vi "Project (1).vi"() -> ()   [LabVIEW 2023]
uses:
  <vilib>/Utility/file.llb/Read Delimited Spreadsheet (string).vi
  <instrlib>/Agilent N934X Series/Agilent N934X Series.lvlib
  System.Windows.Forms
panel:
  out "loop#":i32
  out "size(s)":i32
  out "Trace Data":dbl[](array[numeric])
  in  "Measurement Mode (0: Off)":i32(ring) items=["Off", "Channel Power Measurement", "Adjacent Channel Power Ratio Measurement", "Occupied Bandwidth Measurement", "Spectrum Monitor", "Spectrum Emission Mask", "Channel Scanner", "AM Measurement", "ASK Measurement", "FM Measurement", "FSK Measurement"]
  in  "Measurement Type (0: Spectrum Analyzer)":i32(ring) items=["Spectrum Analyzer", "Tracking Generator", "Power Meter", "Modulation Analyzer", "Reflection Measurement"]
  out "Instrument Firmware Revision":string
  out "Instrument Driver Revision":string
  in  "VISA resource name":refnum<visa-resource-name>
  in  "jkjk":bool
  out "jkjk":string
  out "jkjk":string
  out "jkjk":string
  in  "jkjk":bool
  in  "Tab Control":T1(tab)
  in  "?":bool
  out "?":string
  out "Step:":i32
  in  "Start Frequency (MHz)":dbl
  in  "IIM":bool
  in  "Stop Frequency (MHz)":dbl
  in  "Length of Cable (ft)":dbl
  in  "Cable Attenuation (dB/ft)":dbl
  in  "Velocity Factor (%)":dbl
  out "Waveform Graph":dbl[](graph)
  in  "?":refnum<k24>(container)
  out "Section:":string
  # "VSWR and Distance to Fault Test"
  # "For a single carrier"
  # "(LBand TX)  +  LBand RX = 2475 MHz"
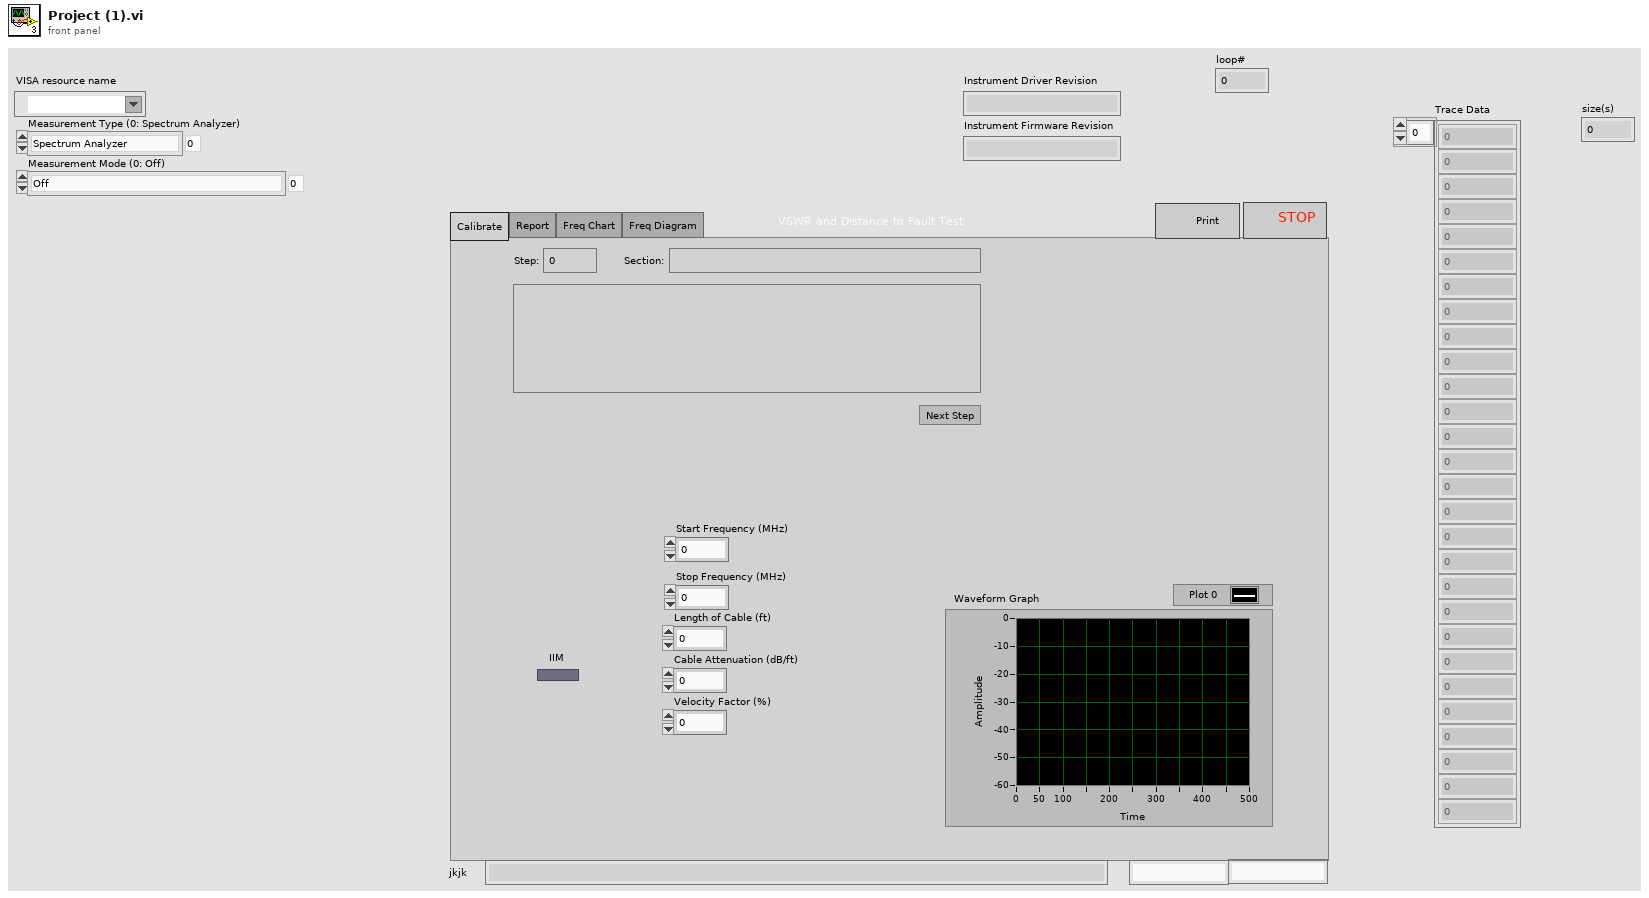
[diagram p1: front panel]
types:
  T1 = enum32{"Calibrate", "Report", "Freq Chart", "Freq Diagram"}
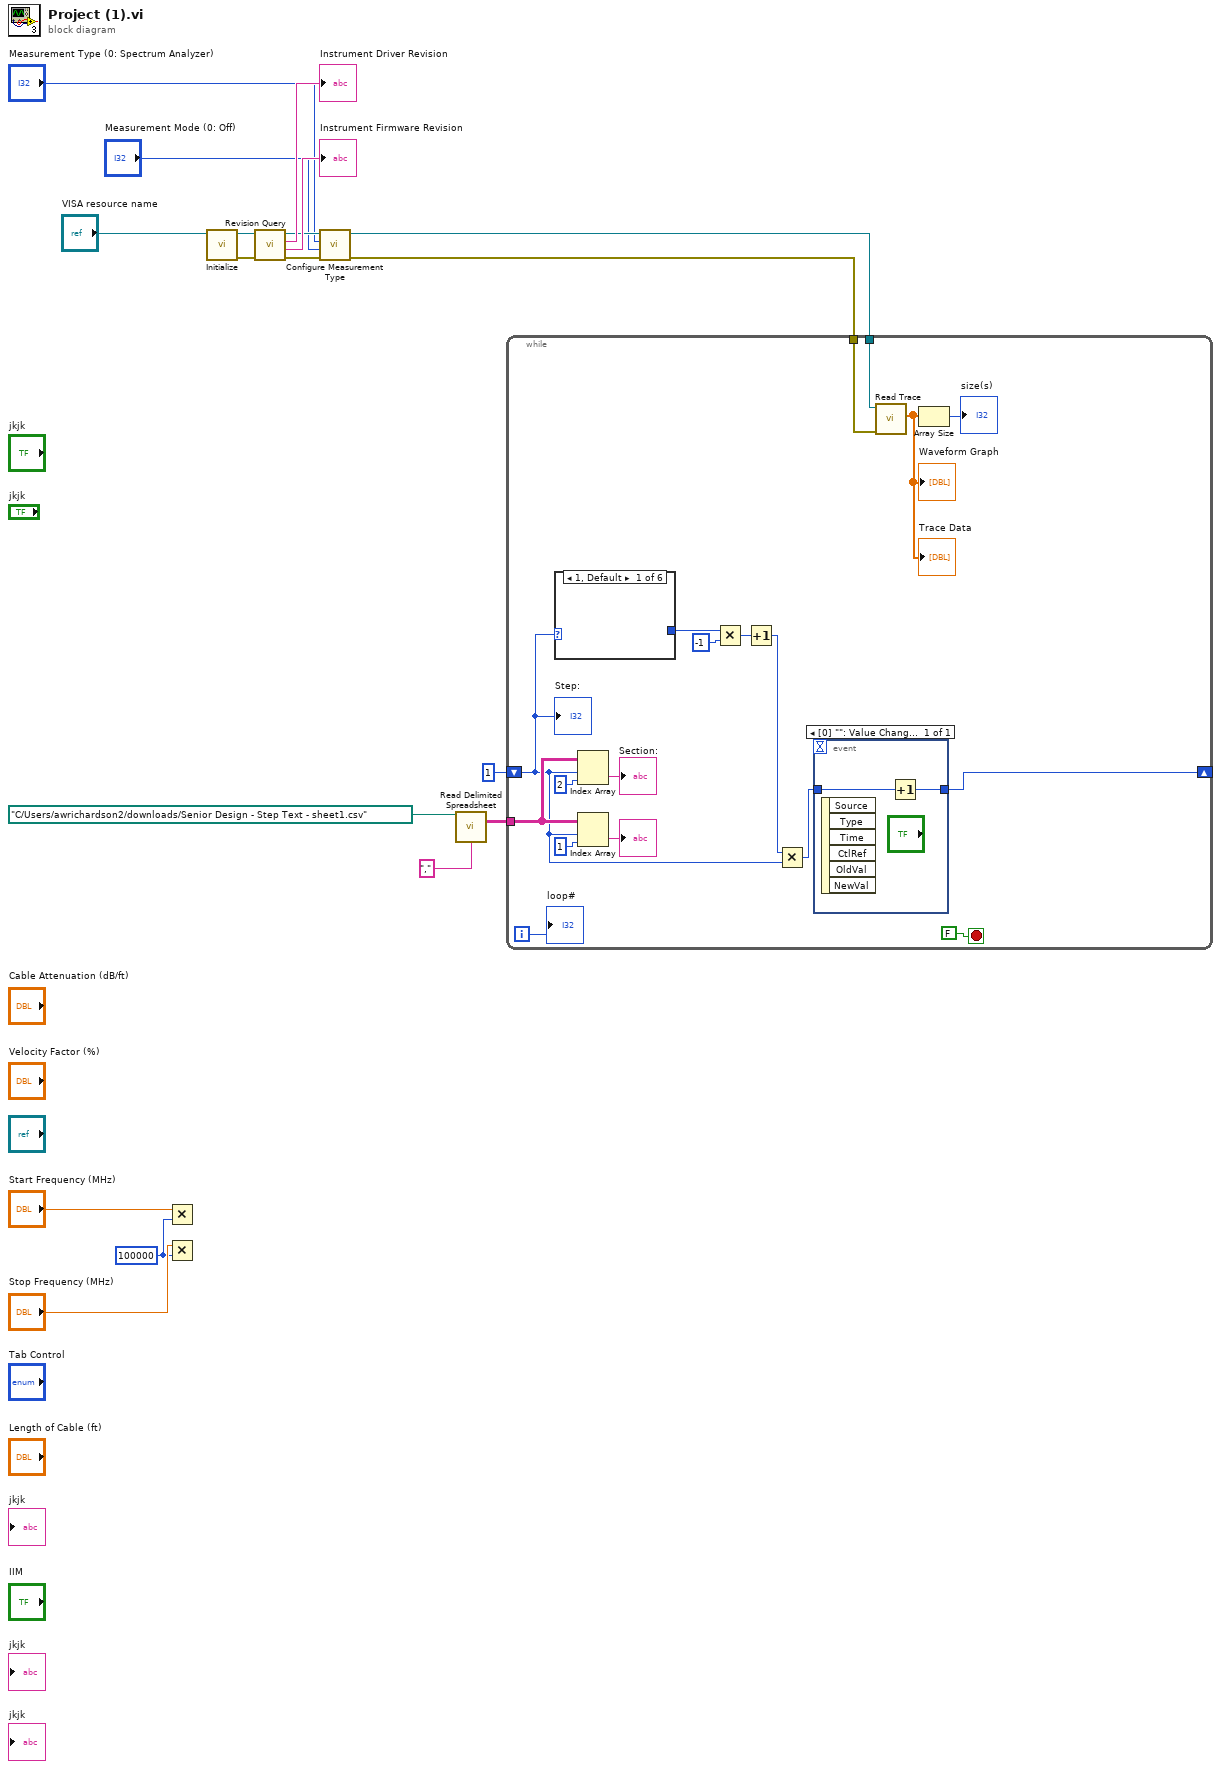
[diagram p0: block diagram]
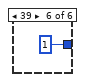
[diagram p6: hidden frame]
diagram:
  w15 = 100000
  n1 = Multiply(x="Start Frequency (MHz)", y=w15) -> ()  [unwired: 1 out]
  n2 = Multiply(x="Stop Frequency (MHz)", y=w15) -> ()  [unwired: 1 out]
  n3 = call <instrlib>:"Initialize.vi"("VISA resource name"="VISA resource name") -> ("error out"=w9:errorcluster, "VISA resource name out"=w10:refnum<visa-resource-name>)  [unwired: 9 in]
  n4 = call <instrlib>:"Revision Query.vi"("error in (no error)"=w9, "VISA resource name"=w10) -> ("error out"=w5:errorcluster, "Instrument Firmware Revision"=→"Instrument Firmware Revision":string, "Instrument Driver Revision"=→"Instrument Driver Revision":string, "VISA resource name out"=w6:refnum<visa-resource-name>)  [unwired: 6 in]
  n5 = call <instrlib>:"Configure Measurement Type.vi"("error in (no error)"=w5, "Measurement Mode (0: Off)"="Measurement Mode (0: Off)", "Measurement Type (0: Spectrum Analyzer)"="Measurement Type (0: Spectrum Analyzer)", "VISA resource name"=w6) -> ("error out"=w2:errorcluster, "VISA resource name out"=w1:refnum<visa-resource-name>)  [unwired: 6 in]
  n6 = call-poly <vilib>:"Read Delimited Spreadsheet.vi"("file path (dialog if empty)"=path "C:/Users/awrichardson2/downloads/Senior Design - Step Text - sheet1.csv", "delimiter (\\t)"="," ("delimiter (\\t)")) -> ("all rows"=w12:string[][])  [unwired: 8 in, 5 out]
  n7 = while {
    shift-right: [w34] -> _
    shift-left: 1 -> [w24]
    tunnel: w12 -> [w26]
    tunnel: w2 -> [w21]
    tunnel: w1 -> [w20]
    i -> [w19]
    stop <- FALSE stop-if-true
    n8 = case shown="1, Default" w24 {
      tunnel: [_ _ _ _ _ 1] -> w33
      frame 1, Default {
      }
      frame 2 {
      }
      frame 3 {
      }
      frame 4 {
      }
      frame 5 {
      }
      frame 39 {
      }
    }
    n9 = Index Array(array=w26, index (row)=w24, index (col)=2) -> (element=→"Section:":string)
    n10 = Index Array(array=w26, index (row)=w24, index (col)=1) -> (element=→"?":string)
    n11 = Multiply(x=w33, y=-1) -> (x*y=w31:i32)
    n12 = Increment(x=w31) -> (x+1=w30:i32)
    n13 = Multiply(x=w30, y=w24) -> (x*y=w35:i32)
    n14 = event shown="[0] \"\": Value Change" {
      selector: _ -> [_]
      dyn-events: _ -> [_]
      timeout: _ -> [_]
      tunnel: w35 -> [w39]
      tunnel: [w38] -> w34
      event Value Change {
        n15 = event-data() -> ()  [unwired: 1 in, 6 out]
        n16 = Increment(x=w39) -> (x+1=w38:i32)
      }
    }
    n17 = call <instrlib>:"Read Trace.vi"("error in (no error)"=w21, "VISA resource name"=w20) -> ("Trace Data"=w23:dbl[])  [unwired: 7 in, 2 out]
    "Waveform Graph" <- w23
    "Trace Data" <- w23
    n18 = Array Size(array=w23) -> (size(s)=→"size(s)":i32)
    "Step:" <- w24
    "loop#" <- w19
  }
